vi "Limit Alarm Client.vi"() -> ()   [LabVIEW 2019, in "OPC UA Demo.lvlib"]
doc: "Demonstrates the use of the <B>OPC UA Alarms and Conditions</B> functionality as an OPC UA Client."
uses:
  OPC UA Demo.lvlib
  <vilib>/OPCUA/controls/NodeIds.ctl
  <vilib>/OPCUA/controls/NodeId.ctl
  <vilib>/OPCUA/NI OPC UA Client.lvlib
panel:
  in  "events view":enum32{"Events", "Alarms", "History Events"}(tab)
  in  "events":i32(listbox)=-1
  in  "acknowledge":bool
  in  "alarms":i32(listbox)=-1
  in  "confirm":bool
  in  "notifier node ID":string="ns=2;s=Level Alarm Notifier"
  in  "start time":timestamp
  in  "history events":i32(listbox)=-1
  in  "end time":timestamp
  in  "history event read":bool
  in  "stop":bool
  in  "auto acknowledge and confirm":bool
  in  "server endpoint URL":string="opc.tcp://localhost:49580"
  # "Overview: Demonstrates the use of the OPC UA Alarms and Conditions functionality as an OPC UA Client.\nRequirements: \n1. LabVIEW OPC UA Toolkit\n2. Run this VI on RT targets or Windows\nInstructions:\n1. Specify the server endpoint URL generated by the server.\n2. Run the VI.\n3. Click the auto acknowledge and confirm to choose whether this VI automatically acknowledges and confirms the condition."
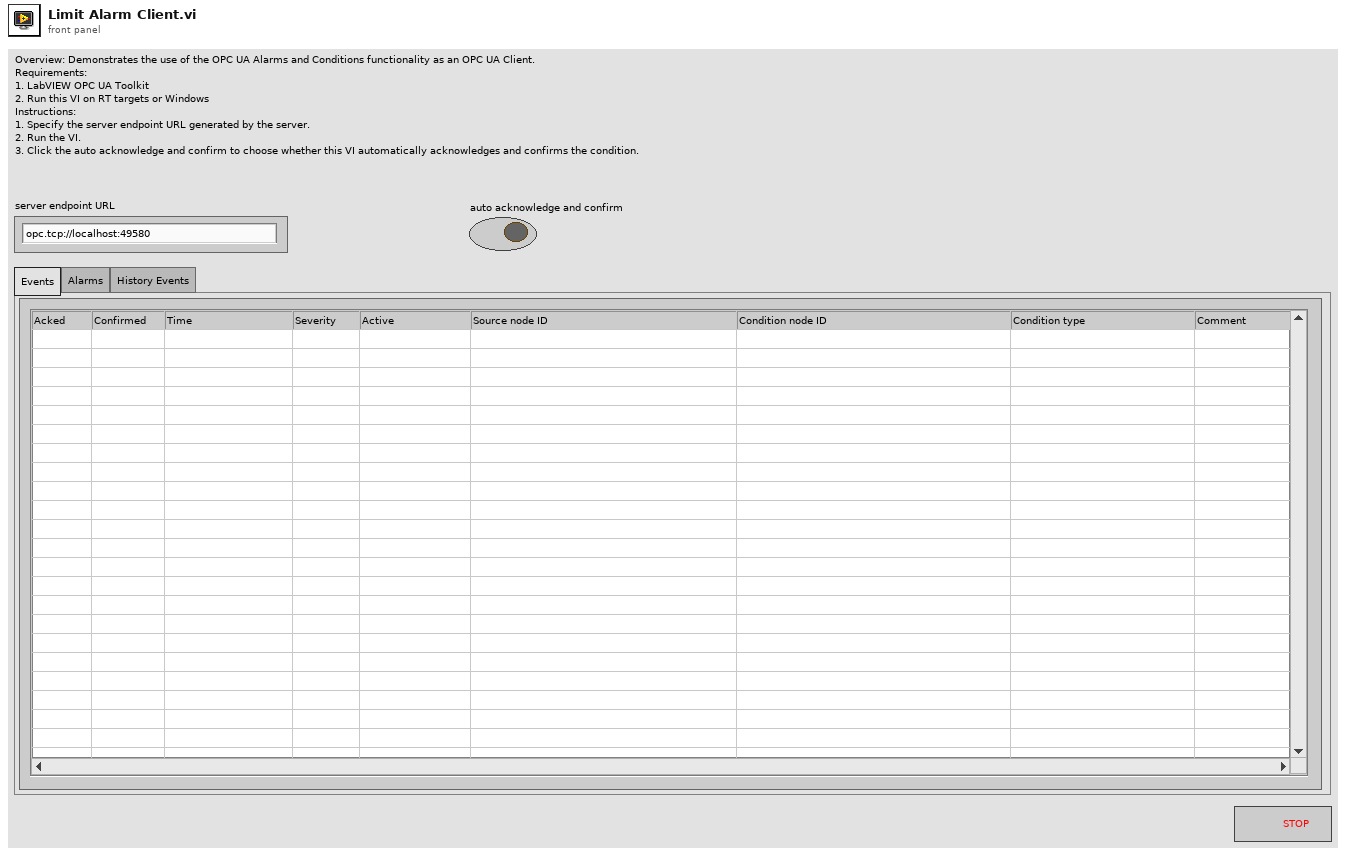
[diagram p1: front panel]
types:
  T1 = typedef "NodeIds.ctl" = T2[]
  T2 = typedef "NodeId.ctl" = string
  T3 = typedef "OPC UA Client Refnum.ctl" = refnum<k21>
  T4 = typedef "Subscription ID.ctl" = u32
  T5 = cluster{"method":u32, "event ID":string, "comment":string}
  T6 = cluster{"continuation point":variant, "has continuation point?":bool}[]
  T7 = cluster{"start time":timestamp, "end time":timestamp, "num values per node":u32}
  T8 = typedef "Event Fields.ctl" = cluster{"condition node ID":T2, "condition type":T9, "source node ID/input node ID":T2, "event ID":string, "active":bool, "time":timestamp, "severity":u16, "quality":T10, "comment":string, "limit state":cluster{"high high state":bool, "high state":bool, "low state":bool, "low low state":bool}, "acked state":bool, "confirmed state":bool, "prompt":string}
  T9 = typedef "Condition Type.ctl" = enum16{"Dialog Condition", "Off-Normal Alarm", "Exclusive Level Alarm", "Exclusive Deviation Alarm", "Exclusive Rate of Change Alarm", "Nonexclusive Level Alarm", "Nonexclusive Deviation Alarm", "Nonexclusive Rate of Change Alarm", "Refresh Start Event", "Refresh End Event"}
  T10 = typedef "OPC UA StatusCode.ctl" = u32
  T11 = typedef "Event Data.ctl" = cluster{"notifier node ID":T2, "history events":T8[], "status":T10}
  T12 = cluster{"continuation point":variant, "has continuation point?":bool}
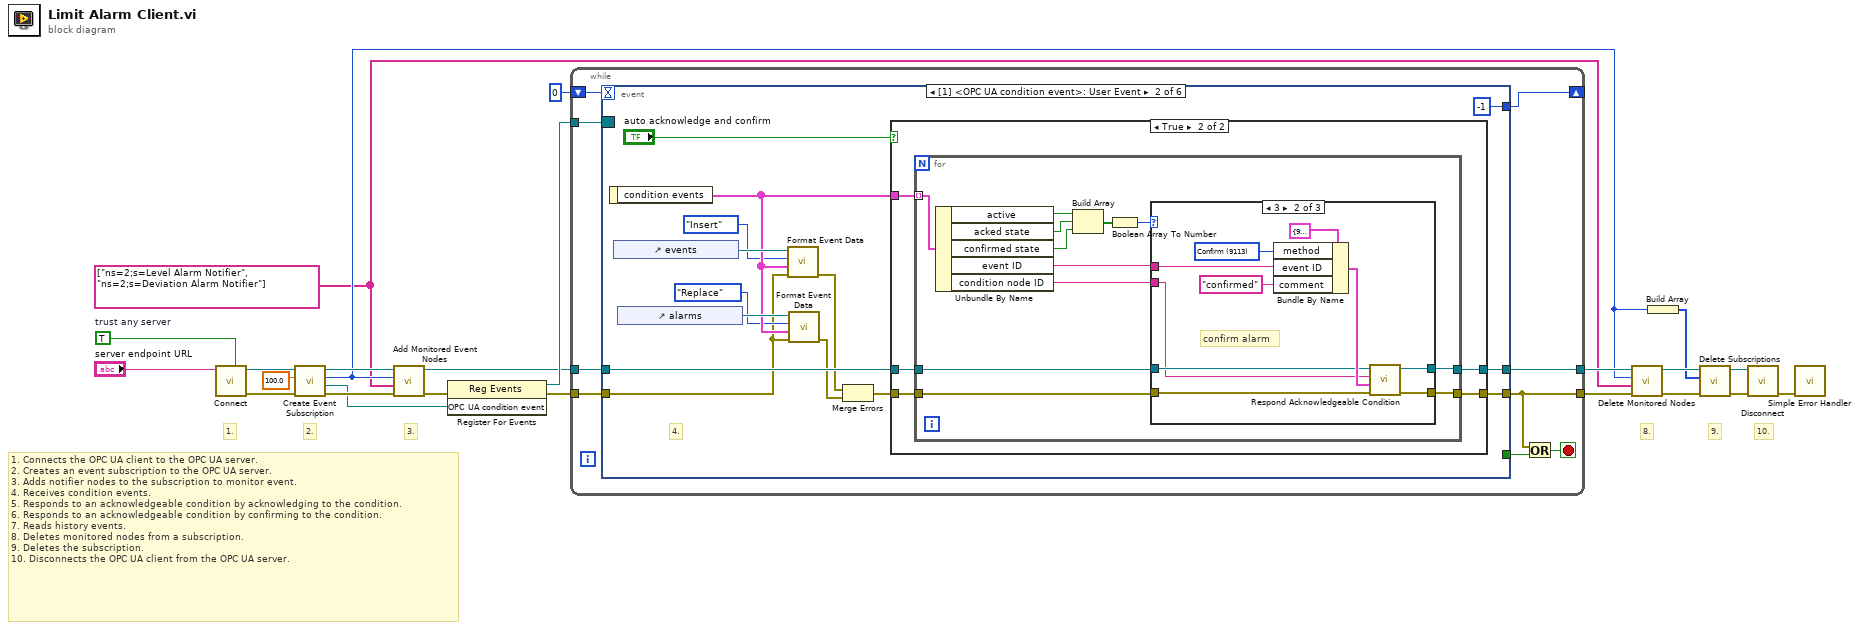
[diagram p0: block diagram]
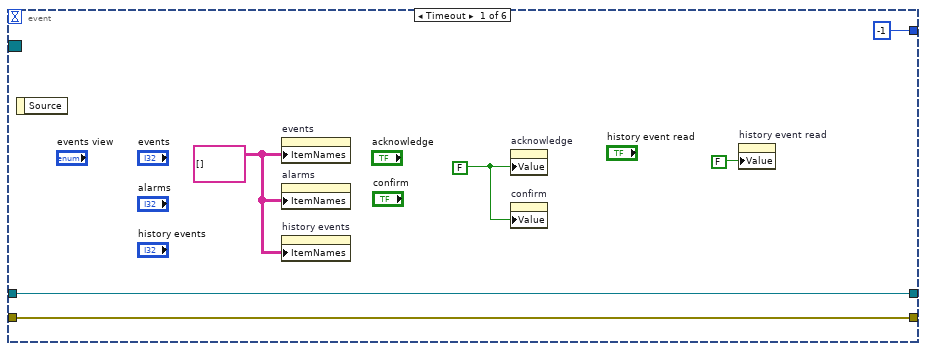
[diagram p2: hidden frame]
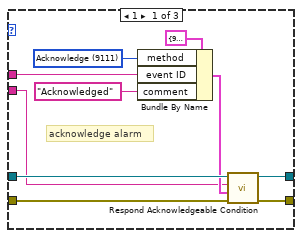
[diagram p4: hidden frame]
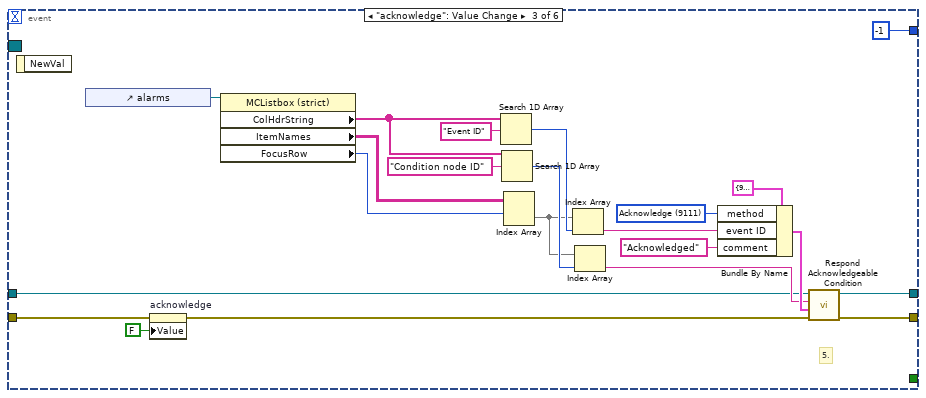
[diagram p6: hidden frame]
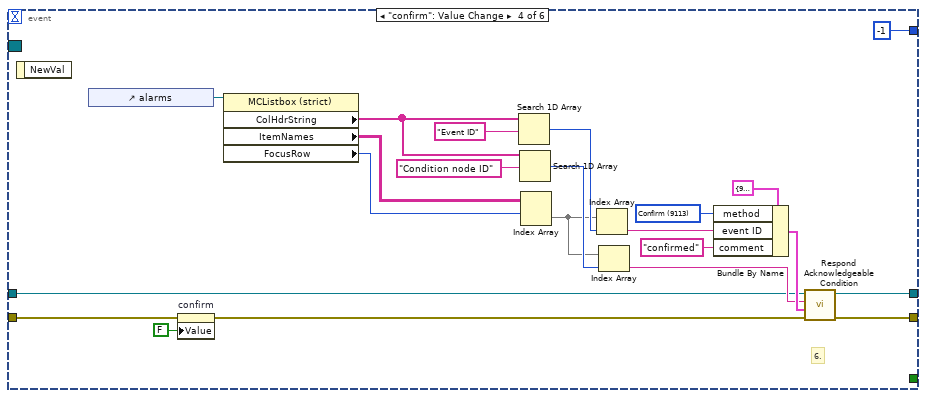
[diagram p7: hidden frame]
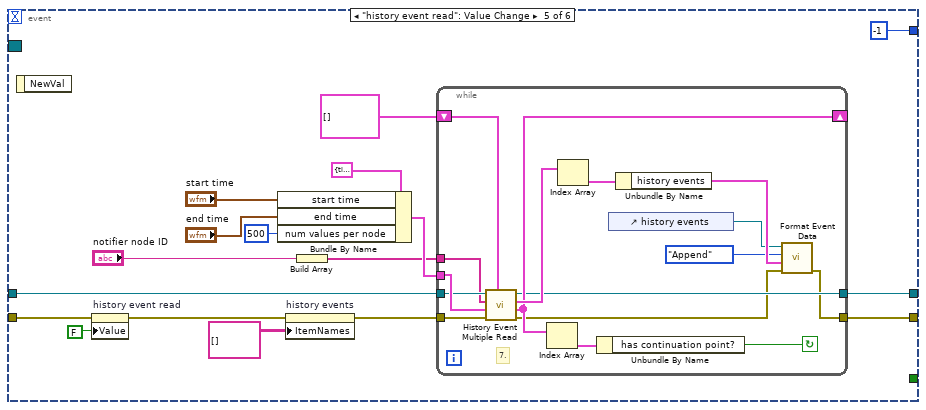
[diagram p8: hidden frame]
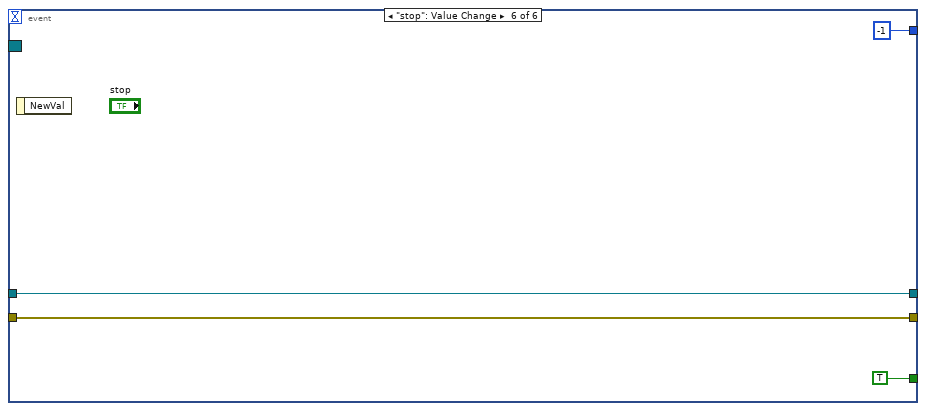
[diagram p9: hidden frame]
diagram:
  w1 = TRUE  # trust any server
  w4 = T1 ["ns=2;s=Level Alarm Notifier", "ns=2;s=Deviation Alarm Notifier"] ("node IDs")
  # "9."
  # "8."
  # "10."
  # "3."
  # "2."
  # "1."
  # "1. Connects the OPC UA client to the OPC UA server. \n2. Creates an event subscription to the OPC UA server.\n3. Adds notifier nodes to the subscription to monitor event.\n4. Receives condition events.\n5. Responds to an acknowledgeable condition by acknowledging to the condition. \n6. Responds to an acknowledgeable condition by confirming to the condition. \n7. Reads history events. \n8. Deletes monitored nodes from a subscription.\n9. Deletes the subscription. \n10. Disconnects the OPC UA client from the OPC UA server."
  n1 = call <vilib>:"Connect.vi"("trust any server (F)"=w1, "server endpoint URL"="server endpoint URL") -> ("error out"=w19:errorcluster, "OPC UA client refnum out"=w18:T3)  [unwired: 7 in, 1 out]
  n2 = call <vilib>:"Create Event Subscription.vi"("error in (no error)"=w19, "publishing interval (1000 ms)"=100.0 ("update rate (1000 ms)"), "OPC UA client refnum in"=w18) -> ("error out"=w23:errorcluster, "OPC UA condition event"=w17:refnum<user-event>, "subscription ID out"=w6:T4, "OPC UA client refnum out"=w22:T3)  [unwired: 4 in, 1 out]
  n3 = call <vilib>:"Add Monitored Event Nodes.vi"("error in (no error)"=w23, "node IDs"=w4, "subscription ID in"=w6, "OPC UA client refnum in"=w22) -> ("error out"=w21:errorcluster, "OPC UA client refnum out"=w13:T3)  [unwired: 4 in, 2 out]
  n4 = register-events(error in=w21, w17) -> (reference out=w15:refnum<event-registration>, error out=w14:errorcluster)  [unwired: 1 in]
  n5 = while {
    tunnel: w15 -> [w32]
    tunnel: w14 -> [w31]
    tunnel: [w25] -> w11
    tunnel: w13 -> [w30]
    tunnel: [w29] -> w12
    shift-right: [w27] -> _
    shift-left: 0 -> [w28]
    stop <- w24 stop-if-true
    n6 = event shown="[1] <OPC UA condition event>: User Event" {
      selector: w32 -> [_ _ _ _ _ _]
      dyn-events: _ -> [_ _ _ _ _ _]
      timeout: w28 -> [_ _ _ _ _ _]
      tunnel: w31 -> [w34 w42 w95 w119 w141 w173]
      tunnel: [w34 w50 w97 w117 w139 w173] -> w25
      tunnel: w30 -> [w35 w52 w96 w120 w142 w174]
      tunnel: [w35 w51 w98 w118 w140 w174] -> w29
      tunnel: [-1 -1 -1 -1 -1 -1] -> w27
      tunnel: [_ _ _ _ _ TRUE] -> w26
      event Timeout {
        w37 = FALSE
        w38 = string[][] [] ("Item Names")
        n7 = event-data() -> ()  [unwired: 1 in, 1 out]
        n8 = property on="events" class="MCListbox (strict)"("ItemNames"=w38) -> ()  [unwired: 2 in, 2 out]
        n9 = property on="alarms" class="MCListbox (strict)"("ItemNames"=w38) -> ()  [unwired: 2 in, 2 out]
        n10 = property on="history events" class="MCListbox (strict)"("ItemNames"=w38) -> ()  [unwired: 2 in, 2 out]
        n11 = property on="acknowledge" class="Bool (strict)"("Value"=w37) -> ()  [unwired: 2 in, 2 out]
        n12 = property on="confirm" class="Bool (strict)"("Value"=w37) -> ()  [unwired: 2 in, 2 out]
        n13 = property on="history event read" class="Bool (strict)"("Value"=FALSE) -> ()  [unwired: 2 in, 2 out]
      }
      event User Event {
        # "4."
        n14 = event-data() -> ("condition events"=w46:T8[])  [unwired: 1 in]
        n15 = control-ref of="events"() -> (w48:refnum<vi>)
        n16 = control-ref of="alarms"() -> (w47:refnum<vi>)
        n17 = call "Format Event Data.vi"("error in"=w42, "event array"=w46, "type"=enum16{"Insert", "Replace", "Append"}."Insert", "Multicolumn Listbox"=w48) -> ("error out"=w39:errorcluster)  [unwired: 4 in, 3 out]
        n18 = call "Format Event Data.vi"("error in"=w42, "event array"=w46, "type"=enum16{"Insert", "Replace", "Append"}."Replace", "Multicolumn Listbox"=w47) -> ("error out"=w40:errorcluster)  [unwired: 4 in, 3 out]
        n19 = Merge Errors(w39, w40) -> (w41:errorcluster)
        n20 = case shown="True" "auto acknowledge and confirm" {
          tunnel: w46 -> [_ w59]
          tunnel: w52 -> [w54 w58]
          tunnel: w41 -> [w53 w57]
          tunnel: [w54 w56] -> w51
          tunnel: [w53 w55] -> w50
          frame False {
          }
          frame True {
            n21 = for {
              tunnel: w59 -> [w68] mode=indexing
              tunnel: w58 -> [w67]
              tunnel: [w71] -> w56
              tunnel: w57 -> [w66]
              tunnel: [w70] -> w55
              n22 = Unbundle By Name(w68) -> ("active"=w64:bool, "acked state"=w63:bool, "confirmed state"=w62:bool, "event ID"=w69:string, "condition node ID"=w65:T2)
              n23 = Build Array(w64, w63, w62) -> (w61:bool[])
              n24 = Boolean Array To Number(Boolean array=w61) -> (number=w60:u32)
              n25 = case shown="3" w60 {
                tunnel: w67 -> [w81 w87 w93]
                tunnel: w66 -> [w80 w86 w92]
                tunnel: w69 -> [w75 w83 _]
                tunnel: [w77 w85 w93] -> w71
                tunnel: [w76 w84 w92] -> w70
                tunnel: w65 -> [w74 w82 _]
                frame 1 {
                  w72 = u32 9111 items=["Add Comment"=9029, "Acknowledge"=9111, "Confirm"=9113] ("method")
                  # "acknowledge alarm"
                  n26 = Bundle By Name(cluster=T5 {"method"=9029, "event ID"="", "comment"=""} ("request"), "method"=w72, "event ID"=w75, "comment"="Acknowledged") -> (w78:T5)
                  n27 = call <vilib>:"Respond Acknowledgeable Condition.vi"("error in (no error)"=w80, "request"=w78, "condition node ID"=w74, "OPC UA client refnum in"=w81) -> ("error out"=w76:errorcluster, "OPC UA client refnum out"=w77:T3)  [unwired: 5 in, 1 out]
                }
                frame 3 {
                  w91 = u32 9113 items=["Add Comment"=9029, "Acknowledge"=9111, "Confirm"=9113] ("method")
                  # "confirm alarm"
                  n28 = Bundle By Name(cluster=T5 {"method"=9029, "event ID"="", "comment"=""} ("request"), "method"=w91, "event ID"=w83, "comment"="confirmed") -> (w89:T5)
                  n29 = call <vilib>:"Respond Acknowledgeable Condition.vi"("error in (no error)"=w86, "request"=w89, "condition node ID"=w82, "OPC UA client refnum in"=w87) -> ("error out"=w84:errorcluster, "OPC UA client refnum out"=w85:T3)  [unwired: 5 in, 1 out]
                }
                frame Default {
                }
              }
            }
          }
        }
      }
      event "acknowledge": Value Change {
        w99 = u32 9111 items=["Add Comment"=9029, "Acknowledge"=9111, "Confirm"=9113] ("method")
        # "5."
        n30 = event-data() -> ()  [unwired: 1 in, 1 out]
        n31 = control-ref of="alarms"() -> (w115:refnum<vi>)
        n32 = property on="acknowledge" class="Bool (strict)"(error in=w95, "Value"=FALSE ("acknowledge")) -> (error out=w102:errorcluster)  [unwired: 1 in, 1 out]
        n33 = property class="MCListbox (strict)"(reference=w115) -> ("ColHdrString"=w110:string[], "ItemNames"=w114:string[][], "FocusRow"=w113:i32)  [unwired: 1 in, 2 out]
        n34 = Search 1D Array(1D array=w110, element="Event ID") -> (index of element=w111:i32)  [unwired: 1 in]
        n35 = Search 1D Array(1D array=w110, element="Condition node ID") -> (index of element=w108:i32)  [unwired: 1 in]
        n36 = Index Array(array=w114, index (row)=w113) -> (element=w104:string[])  [unwired: 1 in]
        n37 = Index Array(array=w104, index=w111) -> (element=w105:string)
        n38 = Index Array(array=w104, index=w108) -> (element=w103:string)
        n39 = Bundle By Name(cluster=T5 {"method"=9029, "event ID"="", "comment"=""} ("request"), "method"=w99, "event ID"=w105, "comment"="Acknowledged") -> (w106:T5)
        n40 = call <vilib>:"Respond Acknowledgeable Condition.vi"("error in (no error)"=w102, "request"=w106, "condition node ID"=w103, "OPC UA client refnum in"=w96) -> ("error out"=w97:errorcluster, "OPC UA client refnum out"=w98:T3)  [unwired: 5 in, 1 out]
      }
      event "confirm": Value Change {
        w121 = u32 9113 items=["Add Comment"=9029, "Acknowledge"=9111, "Confirm"=9113] ("method")
        # "6."
        n41 = event-data() -> ()  [unwired: 1 in, 1 out]
        n42 = control-ref of="alarms"() -> (w137:refnum<vi>)
        n43 = property on="confirm" class="Bool (strict)"(error in=w119, "Value"=FALSE ("confirm")) -> (error out=w124:errorcluster)  [unwired: 1 in, 1 out]
        n44 = property class="MCListbox (strict)"(reference=w137) -> ("ColHdrString"=w132:string[], "ItemNames"=w136:string[][], "FocusRow"=w135:i32)  [unwired: 1 in, 2 out]
        n45 = Search 1D Array(1D array=w132, element="Event ID") -> (index of element=w133:i32)  [unwired: 1 in]
        n46 = Search 1D Array(1D array=w132, element="Condition node ID") -> (index of element=w131:i32)  [unwired: 1 in]
        n47 = Index Array(array=w136, index (row)=w135) -> (element=w127:string[])  [unwired: 1 in]
        n48 = Index Array(array=w127, index=w133) -> (element=w128:string)
        n49 = Index Array(array=w127, index=w131) -> (element=w126:string)
        n50 = Bundle By Name(cluster=T5 {"method"=9029, "event ID"="", "comment"=""} ("request"), "method"=w121, "event ID"=w128, "comment"="confirmed") -> (w129:T5)
        n51 = call <vilib>:"Respond Acknowledgeable Condition.vi"("error in (no error)"=w124, "request"=w129, "condition node ID"=w126, "OPC UA client refnum in"=w120) -> ("error out"=w117:errorcluster, "OPC UA client refnum out"=w118:T3)  [unwired: 5 in, 1 out]
      }
      event "history event read": Value Change {
        n52 = event-data() -> ()  [unwired: 1 in, 1 out]
        n53 = property on="history event read" class="Bool (strict)"(error in=w141, "Value"=FALSE) -> (error out=w143:errorcluster)  [unwired: 1 in, 1 out]
        n54 = Bundle By Name(cluster=T7 {"start time"=timestamp(0 s since 1904-01-01), "end time"=timestamp(0 s since 1904-01-01), "num values per node"=0} ("request"), "start time"="start time", "end time"="end time", "num values per node"=u32 500) -> (w151:T7)
        n55 = property on="history events" class="MCListbox (strict)"(error in=w143, "ItemNames"=string[][] [] ("Item Names")) -> (error out=w146:errorcluster)  [unwired: 1 in, 1 out]
        n56 = Build Array("notifier node ID") -> (w150:string[])
        n57 = while {
          tunnel: w150 -> [w161]
          tunnel: w151 -> [w166]
          tunnel: [w160] -> w140
          tunnel: [w155] -> w139
          shift-right: [w164] -> _
          shift-left: T6 [] ("continuation points in") -> [w165]
          tunnel: w146 -> [w163]
          tunnel: w142 -> [w162]
          stop <- w167 continue-if-true
          # "7."
          n58 = call <vilib>:"History Event Multiple Read.vi"("continuation points in"=w165, "error in (no error)"=w163, "request"=w166, "notifier node IDs"=w161, "OPC UA client refnum in"=w162) -> ("error out"=w156:errorcluster, "continuation points out"=w164:T6, "results"=w170:T11[], "OPC UA client refnum out"=w160:T3)  [unwired: 2 in, 1 out]
          n59 = Index Array(array=w164) -> (element=w168:T12)  [unwired: 1 in]
          n60 = Index Array(array=w170) -> (element=w169:T11)  [unwired: 1 in]
          n61 = Unbundle By Name(w168) -> ("has continuation point?"=w167:bool)
          n62 = control-ref of="history events"() -> (w157:refnum<vi>)
          n63 = Unbundle By Name(w169) -> ("history events"=w159:T8[])
          n64 = call "Format Event Data.vi"("error in"=w156, "event array"=w159, "type"=enum16{"Insert", "Replace", "Append"}."Append", "Multicolumn Listbox"=w157) -> ("error out"=w155:errorcluster)  [unwired: 4 in, 3 out]
        }
      }
      event "stop": Value Change {
        n65 = event-data() -> ()  [unwired: 1 in, 1 out]
      }
    }
    n66 = Or(x=w25, y=w26) -> (x .or. y?=w24:bool)
  }
  n67 = call <vilib>:"Delete Monitored Nodes.vi"("error in (no error)"=w11, "node IDs"=w4, "subscription ID in"=w6, "OPC UA client refnum in"=w12) -> ("error out"=w9:errorcluster, "OPC UA client refnum out"=w10:T3)  [unwired: 3 in, 3 out]
  n68 = Build Array(w6) -> (w7:T4[])
  n69 = call <vilib>:"Delete Subscriptions.vi"("error in (no error)"=w9, "subscription IDs"=w7, "OPC UA client refnum in"=w10) -> ("error out"=w3:errorcluster, "OPC UA client refnum out"=w8:T3)  [unwired: 6 in, 1 out]
  n70 = call <vilib>:"Disconnect.vi"("error in (no error)"=w3, "OPC UA client refnum in"=w8) -> ("error out"=w2:errorcluster)  [unwired: 9 in]
  n71 = call <vilib>:"Simple Error Handler.vi"("error in (no error)"=w2) -> ()  [unwired: 4 in, 5 out]
